vi "Unpack Shortcut Menu Selection.vi"(11 "ShortcutMenuSelectionMsg":refnum<class "ShortcutMenuSelectionMsg.lvclass">) -> (0 "Item Path":string, 1 "Item Tag":string, 2 "Time":u32, 3 "CtlRef":refnum<vi>, 4 "Coords":T1, 5 "Control Label":string, 6 "SubObj":refnum<vi>, 7 "App Item?":bool)   [LabVIEW 2020, in "ActorEvents.lvlib" / "ShortcutMenuSelectionMsg.lvclass"]
doc: "<License>\nCopyright © 2017 Composed Systems, LLC | All rights reserved\nwww.composed.io\n\nAuthor: Ethan Stern <ethan.stern@composed.io>\n\nThis software is provided \"AS IS\" WITHOUT WARRANTIES, either express or implied, AND IS FOR EDUCATIONAL PURPOSES ONLY.\n</License>"
uses:
  <vilib>/gpm_packages/@cs/mva-viewable/Source/ActorEvents/IEventAggregator Messages/ShortcutMenuSelectionMsg/ShortcutMenuSelectionMsg.lvclass
  <vilib>/Utility/miscctls.llb/LVPoint32TypeDef.ctl
  <vilib>/gpm_packages/@cs/mva-viewable/Source/ActorEvents/IEventAggregator Messages/ShortcutMenuSelectionMsg/ShortcutMenuSelectionMsg.lvclass/ShortcutMenuSelectionMsg.ctl
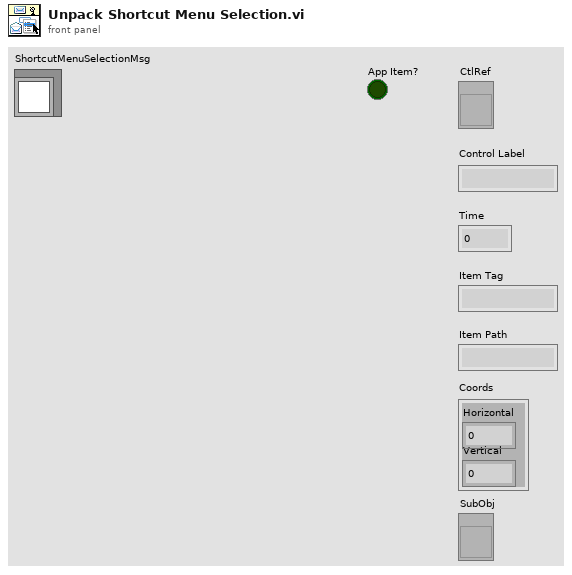
[diagram p1: front panel]
types:
  T1 = typedef "LVPoint32TypeDef.ctl" = cluster{"Horizontal":i32, "Vertical":i32}
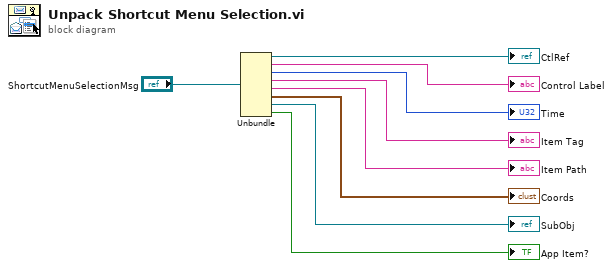
[diagram p0: block diagram]
diagram:
  n1 = Unbundle("ShortcutMenuSelectionMsg") -> (→"CtlRef":refnum<vi>, →"Control Label":string, →"Time":u32, →"Item Tag":string, →"Item Path":string, →"Coords":T1, →"SubObj":refnum<vi>, →"App Item?":bool)
